vi "Install Keyboard Filter.vi"(8 "error in (no error)":errorcluster, 10 "disable <Ctrl>+<Esc> (F)":bool, 11 "disable <Alt>+<Tab> (T)":bool=TRUE) -> (0 "error out":errorcluster)   [LabVIEW 2023, in "WINKEY.lvlib"]
doc: "DOES NOT FUNCTION IN WIN32."
uses:
  WINKEY.lvlib
panel:
  in  "Boolean":bool
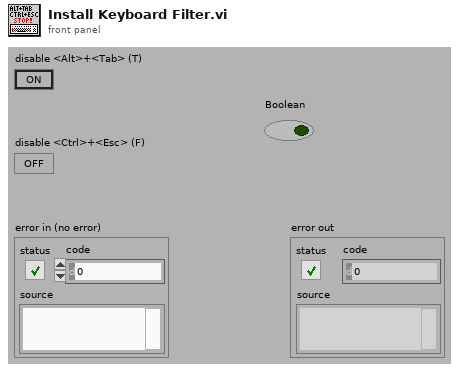
[diagram p1: front panel]
types:
  T1 = cluster{"disable <Ctrl>+<Esc> (F)":bool, "disable <Alt>+<Tab> (T)":bool}
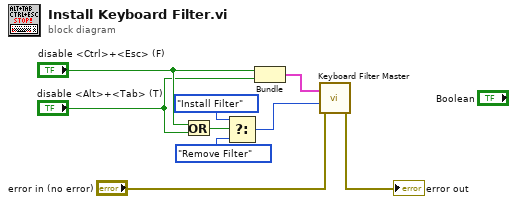
[diagram p0: block diagram]
diagram:
  n1 = Or(x="disable <Ctrl>+<Esc> (F)", y="disable <Alt>+<Tab> (T)") -> (x .or. y?=w6:bool)
  n2 = Select(t=enum16{"Install Filter", "Remove Filter"}."Install Filter", s=w6, f=enum16{"Install Filter", "Remove Filter"}."Remove Filter") -> (s? t:f=w3:enum16{"Install Filter", "Remove Filter"})
  n3 = Bundle("disable <Ctrl>+<Esc> (F)"="disable <Ctrl>+<Esc> (F)", "disable <Alt>+<Tab> (T)"="disable <Alt>+<Tab> (T)") -> (w9:T1)  [unwired: 1 out]
  n4 = call "Keyboard Filter Master.vi"("error in (no error)"="error in (no error)", "install / remove filter"=w3, "filter types"=w9) -> ("error out"=→"error out":errorcluster)  [unwired: 2 out]
